vi "Begin.vi"(8 "error in (no error)":errorcluster, 11 "Pressure in":refnum<class "Pressure.lvclass">) -> (0 "error out":errorcluster, 3 "Pressure out":refnum<class "Pressure.lvclass">)   [LabVIEW 2014, in "Pressure.lvlib" / "Pressure.lvclass"]
uses:
  Pressure.lvclass
  <vilib>/ActorFramework/Actor/Actor.lvclass/Actor.ctl
  <vilib>/ActorFramework/Message Enqueuer/Message Enqueuer.lvclass/Message Enqueuer.ctl
  <vilib>/ActorFramework/Message Enqueuer/Init from Existing Queue.vi
  <vilib>/ActorFramework/Message Enqueuer/Enqueue.vi
  <vilib>/ActorFramework/Message Priority Queue/Priority Enqueue.vi
  Robot Actor Framework/System Actor/System Actor Class/System Actor.lvclass
  <vilib>/ActorFramework/Message Enqueuer/Message Enqueuer.lvclass
  Pressure Messages/Enable Msg/Enable Msg.lvclass
  <vilib>/ActorFramework/Actor/Actor.lvclass
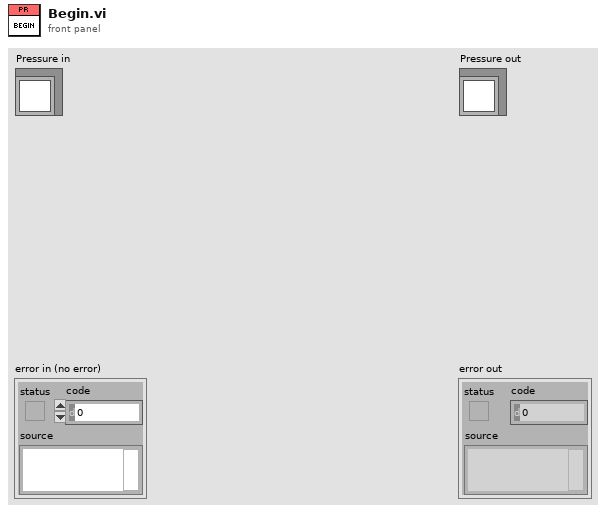
[diagram p1: front panel]
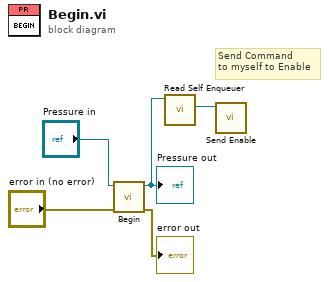
[diagram p0: block diagram]
diagram:
  # "Send Command \nto myself to Enable"
  n1 = call-parent "Begin.vi"("error in (no error)"="error in (no error)", "System Actor in"="Pressure in") -> ("error out"=→"error out":errorcluster, "System Actor out"=w2:refnum<class "Pressure.lvclass">)  [unwired: 8 in]
  "Pressure out" <- w2
  n2 = call <vilib>:"Read Self Enqueuer.vi"("Actor"=w2) -> ("Self Enqueuer"=w1:refnum<class "Message Enqueuer.lvclass">)  [unwired: 10 in]
  n3 = call "Send Enable.vi"("Message Enqueuer"=w1) -> ()  [unwired: 9 in, 2 out]
